vi "Eval Single-Variable Scalar.vi"(2 "error in (no error)":errorcluster, 3 "x value":dbl format="%0.2f", 4 "formula":string) -> (0 "error out":errorcluster, 1 "y value":dbl format="%0.2f")   [LabVIEW 2017, in "NI_Gmath.lvlib"]
doc: "Calculates exactly one function value of a given 1D function y = f(x), where f is the function specified by the user formula."
uses:
  NI_Gmath.lvlib
panel:
  # "Example:\n\n formula: x*sin(x) \n x value: 1.56"
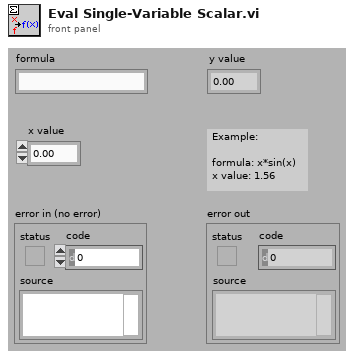
[diagram p1: front panel]
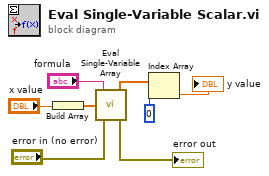
[diagram p0: block diagram]
diagram:
  n1 = Build Array("x value") -> (w3:dbl[])
  n2 = call "Eval Single-Variable Array.vi"("error in (no error)"="error in (no error)", "X Values"=w3, "formula"="formula") -> ("error out"=→"error out":errorcluster, "Y Values"=w8:dbl[])
  n3 = Index Array(array=w8, index=0) -> (element=→"y value":dbl)
